vi "Get Current Project.vi"(6 "timeout (ms)":i32=-1, 8 "error in (no error)":errorcluster, 11 "FlexLogger_gRPC in":refnum<class "FlexLogger_gRPC.lvclass">) -> (0 "error out":errorcluster, 2 "Response Data":T1, 3 "FlexLogger_gRPC out":refnum<class "FlexLogger_gRPC.lvclass">)   [LabVIEW 2020, in "FlexLogger_gRPC.lvlib" / "FlexLogger_gRPC.lvclass"]
doc: "Gets the currently active (open) project from the Flexlogger Application."
uses:
  FlexLogger_gRPC.lvclass
  FlexLogger_client/RPC Messages/flexlogger_GetActiveProjectResponse.ctl
  FlexLogger_client/RPC Messages/flexlogger_ProjectIdentifier.ctl
  FlexLogger_gRPC.lvclass/FlexLogger_gRPC.ctl
  FlexLogger_client/FlexLogger_client.lvlib
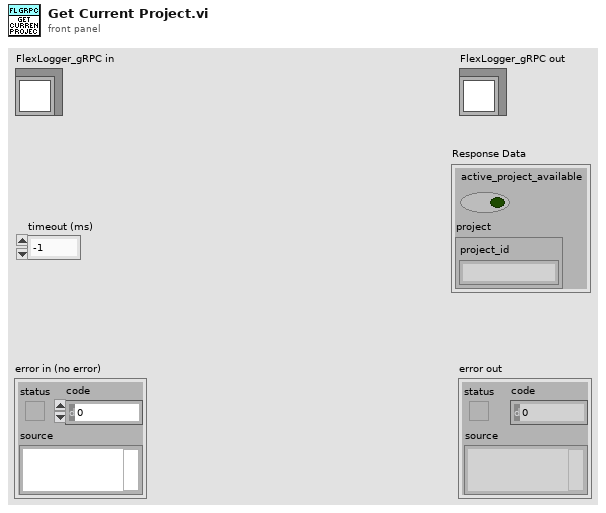
[diagram p1: front panel]
types:
  T1 = typedef "FlexLogger_client.lvlib/flexlogger_GetActiveProjectResponse.ctl" = cluster{"active_project_available":bool, "project":T2}
  T2 = typedef "FlexLogger_client.lvlib/flexlogger_ProjectIdentifier.ctl" = cluster{"project_id":string}
  T3 = typedef "grpc-lvsupport-release.lvlib/grpcId.ctl" = u64
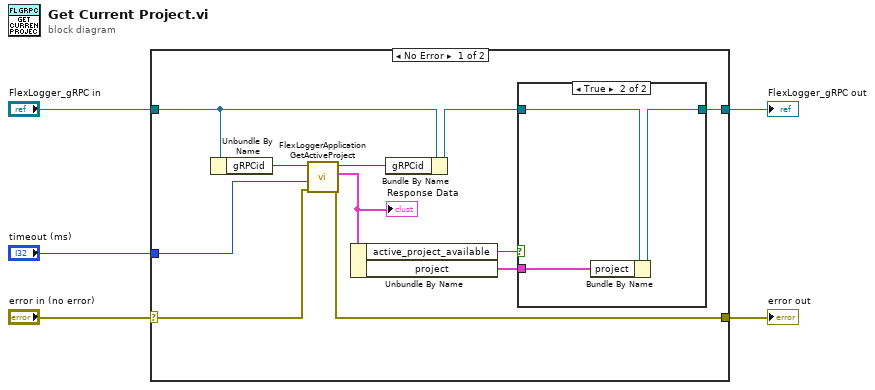
[diagram p0: block diagram]
diagram:
  n1 = case shown="No Error" "error in (no error)" {
    selector: "error in (no error)" -> [w14 w21]
    tunnel: "FlexLogger_gRPC in" -> [w13 w22]
    tunnel: [w9 w22] -> w4
    tunnel: [w11 w21] -> w3
    tunnel: "timeout (ms)" -> [w6 _]
    frame No Error {
      n2 = Unbundle By Name(w13) -> ("gRPCid"=w15:T3)
      n3 = call "FlexLoggerApplication GetActiveProject.vi"("error in"=w14, "timeout (ms)"=w6, "gRPC ID"=w15) -> ("error out"=w11:errorcluster, "Response Data"=w16:T1, "gRPC ID out"=w12:T3)  [unwired: 6 in]
      "Response Data" <- w16
      n4 = Unbundle By Name(w16) -> ("active_project_available"=w7:bool, "project"=w8:T2)
      n5 = Bundle By Name(cluster=w13, "gRPCid"=w12) -> (w10:refnum<class "FlexLogger_gRPC.lvclass">)
      n6 = case shown="True" w7 {
        tunnel: w10 -> [w17 w20]
        tunnel: [w17 w19] -> w9
        tunnel: w8 -> [_ w18]
        frame False {
        }
        frame True {
          n7 = Bundle By Name(cluster=w20, "project"=w18) -> (w19:refnum<class "FlexLogger_gRPC.lvclass">)
        }
      }
    }
    frame Error {
    }
  }
  "error out" <- w3
  "FlexLogger_gRPC out" <- w4
